vi "Write File.vi"(8 "error in (no error)":errorcluster, 11 "[Data] Recent User in":refnum<class "[User] Recent Login.lvclass">) -> (0 "error out":errorcluster, 3 "[Data] Recent User out":refnum<class "[User] Recent Login.lvclass">)   [LabVIEW 2020, in "[User] Recent Login.lvclass"]
uses:
  [User] Recent Login.lvclass
  [User] Recent Login.lvclass/[User] Recent Login.ctl
  <vilib>/YU/YU-Encrypt/Base64/Base64.lvclass
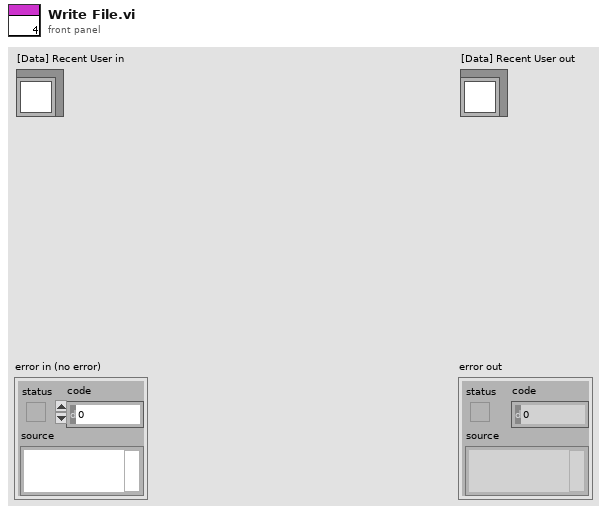
[diagram p1: front panel]
types:
  T1 = enum16{"open", "replace", "create", "open or create", "replace or create", "replace or create with confirmation"}
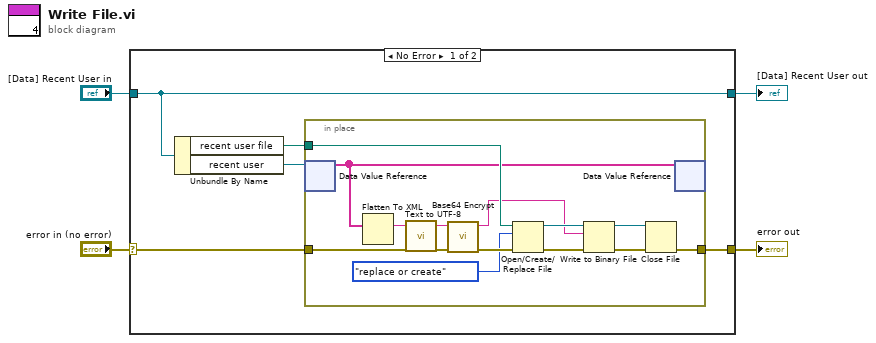
[diagram p0: block diagram]
diagram:
  n1 = case shown="No Error" "error in (no error)" {
    selector: "error in (no error)" -> [w7 w24]
    tunnel: [w5 w24] -> w3
    tunnel: [w9 w23] -> w1
    tunnel: "[Data] Recent User in" -> [w9 w23]
    frame No Error {
      n2 = Unbundle By Name(w9) -> ("recent user file"=w6:path, "recent user"=w8:refnum<data-value>)
      n3 = in-place {
        in-place-border: w7 -> [w10]
        in-place-border: w6 -> [w16]
        in-place-border: [w13] -> w5
        n4 = in-place-dvr #1(w8) -> (w12:string[])  [unwired: 1 out]
        n5 = Flatten To XML(6:w12) -> (2:w11:string)
        n6 = call <vilib>:"Text to UTF-8.vi"("text"=w11) -> ("utf-8 text"=w22:string)  [unwired: 4 in]
        n7 = call <vilib>:"Base64 Encrypt.vi"("error in (no error)"=w10, "data"=w22) -> ("error out"=w17:errorcluster, "encrypted data"=w14:string)  [unwired: 8 in]
        n8 = Open/Create/Replace File(file path (use dialog)=w16, error in=w17, operation (0:open)=T1."replace or create") -> (refnum out=w19:refnum<file>, error out=w18:errorcluster)  [unwired: 3 in, 1 out]
        n9 = Write to Binary File(file (use dialog)=w19, data=w14, error in=w18) -> (refnum out=w21:refnum<file>, error out=w20:errorcluster)  [unwired: 3 in, 1 out]
        n10 = Close File(refnum=w21, error in=w20) -> (error out=w13:errorcluster)  [unwired: 1 out]
        n11 = in-place-dvr #1(w12) -> ()  [unwired: 2 out]
      }
    }
    frame Error {
    }
  }
  "error out" <- w3
  "[Data] Recent User out" <- w1
